vi "DLUpdate-Com-Exec.vi"(8 "error in (no error)":errorcluster, 9 "axisnum refs":refnum<vi>[](array[refnum]), 10 "Axis refs":refnum<vi>[](array[refnum]), 11 "DelayLine.lvclass":refnum<class "DelayLine.lvclass">) -> (0 "error out":errorcluster, 3 "DelayLine out":refnum<class "DelayLine.lvclass">)   [LabVIEW 2019, in "DelayLine.lvclass"]
uses:
  DelayLine.lvclass
  C:/Dev/TRANCON/Classes/GeneralFunctionality/GeneralFunctionality.lvclass
  GeneralFunctionality/GeneralFunctionality.lvclass/GeneralFunctionality.ctl
  GeneralFunctionality/GeneralFunctionality.lvclass
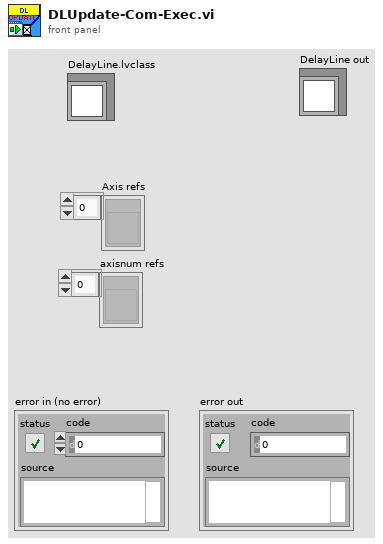
[diagram p1: front panel]
types:
  T1 = enum8{"Enabled", "Disabled", "Disabled and Grayed Out"}
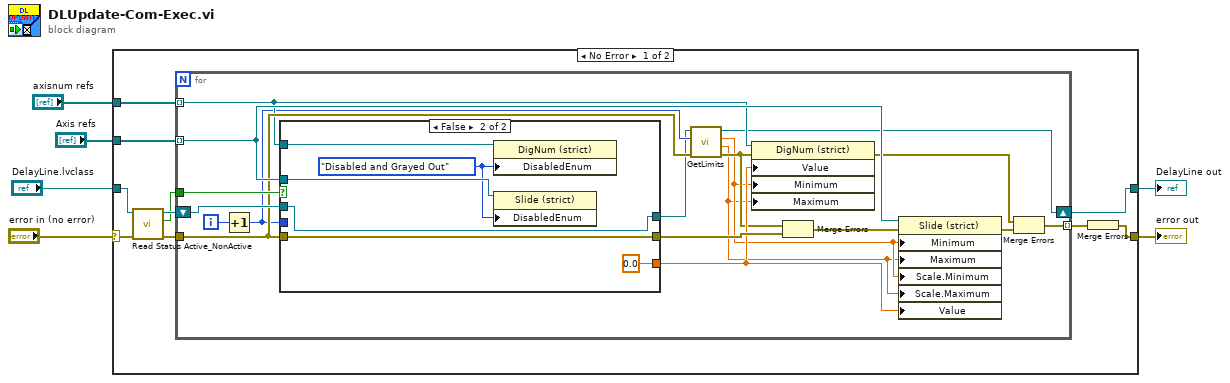
[diagram p0: block diagram]
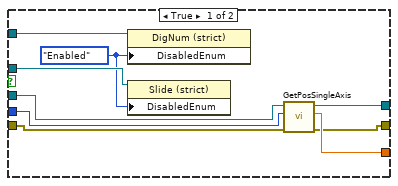
[diagram p2: hidden frame]
diagram:
  n1 = case shown="No Error" "error in (no error)" {
    selector: "error in (no error)" -> [w10 w51]
    tunnel: [w16 w51] -> w6
    tunnel: [w7 w50] -> w5
    tunnel: "DelayLine.lvclass" -> [w11 w50]
    tunnel: "axisnum refs" -> [w9 _]
    tunnel: "Axis refs" -> [w8 _]
    frame No Error {
      n2 = call "Read Status Active_NonActive.vi"("error in (no error)"=w10, "GeneralFunctionality in"=w11) -> ("error out"=w13:errorcluster, "Status Active/NonActive"=w12:bool, "GeneralFunctionality out"=w15:refnum<class "DelayLine.lvclass">)  [unwired: 7 in]
      n3 = for {
        tunnel: w8 -> [w33] mode=indexing
        tunnel: w12 -> [w34]
        tunnel: w13 -> [w30]
        tunnel: [w26] -> w14 mode=indexing
        tunnel: w9 -> [w21] mode=indexing
        shift-right: [w17] -> w7
        shift-left: w15 -> [w31]
        i -> [w20]
        n4 = Increment(x=w20) -> (x+1=w19:i32)
        n5 = case shown="False" w34 {
          tunnel: w33 -> [w43 w49]
          tunnel: w31 -> [w41 w44]
          tunnel: w19 -> [w40 _]
          tunnel: w30 -> [w42 w48]
          tunnel: [w38 w48] -> w29
          tunnel: [w39 0.0 ("Pos")] -> w28
          tunnel: w21 -> [w36 w45]
          tunnel: [w35 w44] -> w18
          frame True {
            w37 = T1."Enabled" ("Désactivé")
            n6 = property class="DigNum (strict)"(reference=w36, "DisabledEnum"=w37) -> ()  [unwired: 1 in, 2 out]
            n7 = property class="Slide (strict)"(reference=w43, "DisabledEnum"=w37) -> ()  [unwired: 1 in, 2 out]
            n8 = call-dynamic "GetPosSingleAxis.vi"("error in (no error)"=w42, "Axis"=w40, "DelayLine in"=w41) -> ("error out"=w38:errorcluster, "Pos"=w39:dbl, "DelayLine out"=w35:refnum<class "DelayLine.lvclass">)  [unwired: 6 in]
          }
          frame False {
            w46 = T1."Disabled and Grayed Out" ("Désactivé")
            n9 = property class="DigNum (strict)"(reference=w45, "DisabledEnum"=w46) -> ()  [unwired: 1 in, 2 out]
            n10 = property class="Slide (strict)"(reference=w49, "DisabledEnum"=w46) -> ()  [unwired: 1 in, 2 out]
          }
        }
        n11 = call-dynamic "GetLimits.vi"("error in (no error)"=w30, "Axis"=w19, "DelayLine in"=w18) -> ("error out"=w24:errorcluster, "max"=w22:dbl, "min"=w23:dbl, "DelayLine out"=w17:refnum<class "DelayLine.lvclass">)  [unwired: 4 in, 1 out]
        n12 = property class="DigNum (strict)"(reference=w21, error in=w24, "Value"=w28, "Minimum"=w23, "Maximum"=w22) -> (error out=w25:errorcluster)  [unwired: 1 out]
        n13 = Merge Errors(w24, w29) -> (w32:errorcluster)
        n14 = property class="Slide (strict)"(reference=w33, error in=w32, "Minimum"=w23, "Maximum"=w22, "Scale.Minimum"=w23, "Scale.Maximum"=w22, "Value"=w28) -> (error out=w27:errorcluster)  [unwired: 1 out]
        n15 = Merge Errors(w25, w27) -> (w26:errorcluster)
      }
      n16 = Merge Errors(w14) -> (w16:errorcluster)
    }
    frame Error {
    }
  }
  "error out" <- w6
  "DelayLine out" <- w5
